vi "UDT_ErrorMonitorModule_ErrorStart.vi"() -> (3 "Unit Test Framework Results":T1)   [LabVIEW 2017]
doc: "Use this template to create a user-defined test VI. Define your test requirements and wire the results to the <b>Result (Test)</b> control. Do not modify the <b>Unit Test Framework Results</b> indicator."
uses:
  <vilib>/utf/common/utf_test_result_troll.ctl
  <vilib>/utf/common/utf_test_result.ctl
  <vilib>/utf/common/utf_test_result_failure.ctl
  <vilib>/utf/common/utf_test_comparison_operators.ctl
  <vilib>/utf/common/utf_vi_tag.ctl
  RT/programControl/StartUEFGV/TypeDefs/UEFGVcontrol.ctl
  RT/TypeDefs/LoopStates.ctl
  <vilib>/Control Software Solutions Ltd/UTF Helper/SubVIs/UTF I32 Equals.vi
  RT/programControl/programControl.lvlib
  RT/communicateMLC/communicateMLC.lvlib
  RT/externalAcquisition/externalAquisition.lvlib
  RT/LowLevelController/lowLevelController.lvlib
  RT/loggingModule/loggingModule.lvlib
  RT/ErrorMonitor/ErrorMonitor.lvlib
  <vilib>/Control Software Solutions Ltd/UTF Helper/Unit Test Helper.lvlib
  <vilib>/utf/NI_UnitTestFramework.lvlib
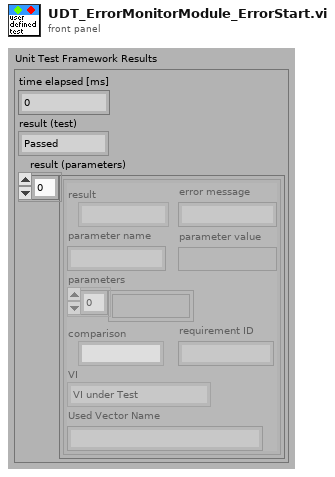
[diagram p1: front panel]
types:
  T1 = typedef "NI_UnitTestFramework.lvlib/utf_test_result_troll.ctl" = cluster{"time elapsed [ms]":u32, "result (test)":T2, "result (parameters)":T3[]}
  T2 = typedef "NI_UnitTestFramework.lvlib/utf_test_result.ctl" = enum16{"Passed", "Failed", "Error", "Skipped", "Not Processed"}
  T3 = typedef "NI_UnitTestFramework.lvlib/utf_test_result_failure.ctl" = cluster{"result":T2, "error message":string, "parameter name":string, "parameter value":variant, "parameters":variant[], "comparison":T4, "requirement ID":string, "VI":T5, "Used Vector Name":string}
  T4 = typedef "NI_UnitTestFramework.lvlib/utf_test_comparison_operators.ctl" = enum16{"=", "!=", ">", ">=", "<", "<=", "range", "symmetric tolerance", "asymmetric tolerance", "string contains", "string not contain", "array size", "string length", "array range", "by element", "array range (limit array)", "user-defined", "array contains", "array not contain", "vector length", "= (elm)", "!= (elm)", "= (case insensitive)", "!= (case insensitive)"}
  T5 = typedef "NI_UnitTestFramework.lvlib/utf_vi_tag.ctl" = enum16{"Setup VI", "VI under Test", "Teardown VI"}
  T6 = typedef "LoopStates.ctl" = enum16{"start", "wait", "run", "end"}
  T7 = typedef "UEFGVcontrol.ctl" = enum16{"Create", "Get", "Destroy"}
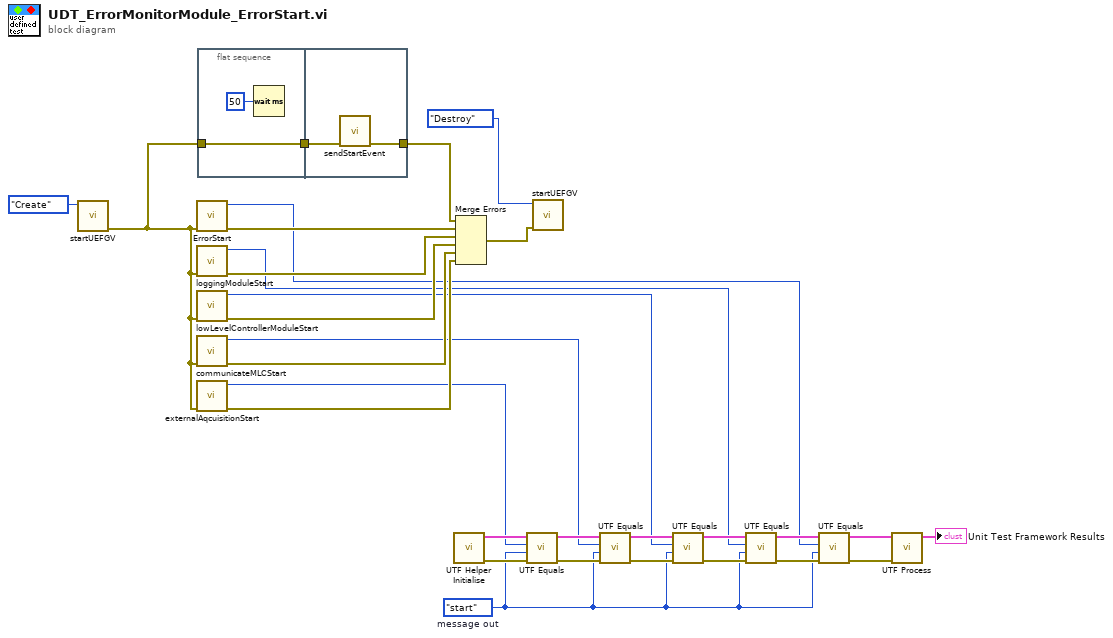
[diagram p0: block diagram]
diagram:
  w4 = LoopStates."start"  # message out
  n1 = call "startUEFGV.vi"("Enum"=UEFGVcontrol."Create") -> ("error out"=w3:errorcluster)  [unwired: 9 in, 1 out]
  n2 = call "ErrorStart.vi"("error in (no error)"=w3) -> ("error out"=w28:errorcluster, "message out"=w5:T6)  [unwired: 9 in]
  n3 = call "loggingModuleStart.vi"("error in (no error)"=w3) -> ("error out"=w24:errorcluster, "message out"=w6:T6)  [unwired: 9 in]
  n4 = call "lowLevelControllerModuleStart.vi"("error in (no error)"=w3) -> ("error out"=w25:errorcluster, "message out"=w7:T6)  [unwired: 9 in]
  n5 = call "communicateMLCStart.vi"("error in (no error)"=w3) -> ("error out"=w26:errorcluster, "message out"=w8:T6)  [unwired: 9 in]
  n6 = call "externalAqcuisitionStart.vi"("error in (no error)"=w3) -> ("error out"=w27:errorcluster, "message out"=w9:T6)  [unwired: 9 in]
  n7 = flat-sequence {
    tunnel: w3 -> [w31]
    tunnel: [w31] -> w30
    tunnel: w30 -> [w34]
    tunnel: [w33] -> w2
    frame #0 {
      n8 = Wait (ms)(milliseconds to wait=u32 50) -> ()  [unwired: 1 out]
    }
    frame #1 {
      n9 = call "sendStartEvent.vi"("error in (no error)"=w34) -> ("error out"=w33:errorcluster)  [unwired: 10 in]
    }
  }
  n10 = call <vilib>:"UTF Helper Initialise.vi"() -> ("error out"=w20:errorcluster, "results array"=w21:T3[])  [unwired: 10 in]
  n11 = Merge Errors(w2, w28, w24, w25, w26, w27) -> (w22:errorcluster)
  n12 = call-poly <vilib>:"UTF Equals.vi"("error in (no error)"=w20, "Test Value"=w4, "Input"=w9, "Input Results"=w21) -> ("error out"=w18:errorcluster, "Output Results"=w19:T3[])  [unwired: 6 in]
  n13 = call "startUEFGV.vi"("error in (no error)"=w22, "Enum"=UEFGVcontrol."Destroy") -> ()  [unwired: 8 in, 2 out]
  n14 = call-poly <vilib>:"UTF Equals.vi"("error in (no error)"=w18, "Test Value"=w4, "Input"=w8, "Input Results"=w19) -> ("error out"=w16:errorcluster, "Output Results"=w17:T3[])  [unwired: 6 in]
  n15 = call-poly <vilib>:"UTF Equals.vi"("error in (no error)"=w16, "Test Value"=w4, "Input"=w7, "Input Results"=w17) -> ("error out"=w14:errorcluster, "Output Results"=w15:T3[])  [unwired: 6 in]
  n16 = call-poly <vilib>:"UTF Equals.vi"("error in (no error)"=w14, "Test Value"=w4, "Input"=w6, "Input Results"=w15) -> ("error out"=w12:errorcluster, "Output Results"=w13:T3[])  [unwired: 6 in]
  n17 = call-poly <vilib>:"UTF Equals.vi"("error in (no error)"=w12, "Test Value"=w4, "Input"=w5, "Input Results"=w13) -> ("error out"=w10:errorcluster, "Output Results"=w11:T3[])  [unwired: 6 in]
  n18 = call <vilib>:"UTF Process.vi"("error in (no error)"=w10, "results array"=w11) -> ("Unit Test Framework Results"=→"Unit Test Framework Results":T1)  [unwired: 9 in]
